vi "OpenG Reverse 2D Array Template.vi"() -> ()   [LabVIEW 2012]
panel:
  in  "by rows or columns (rows)":enum16{"rows", "columns"}(ring)
  in  "Array":dbl[][](array[numeric]) format="%.2f"
  out "Reversed Array":dbl[][](array[numeric]) format="%.2f"
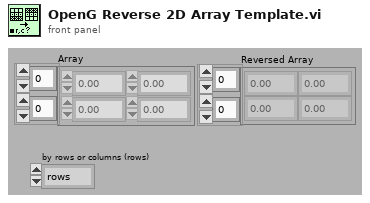
[diagram p1: front panel]
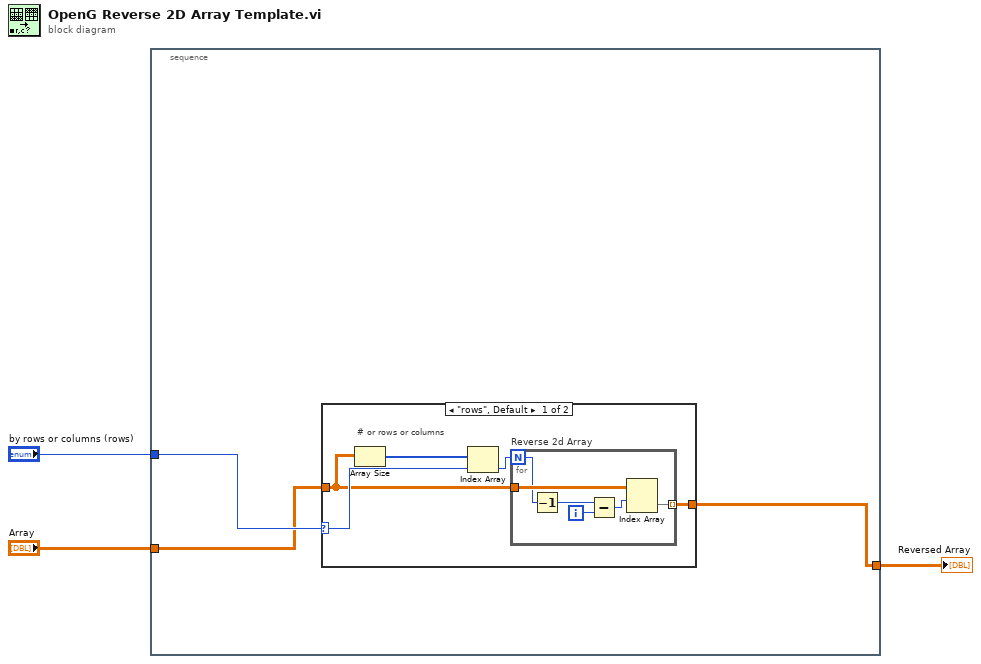
[diagram p0: block diagram]
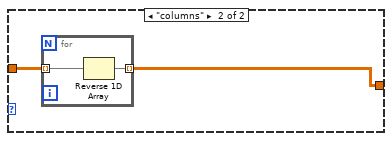
[diagram p2: hidden frame]
diagram:
  n1 = stacked-sequence {
    tunnel: "Array" -> [w5]
    tunnel: "by rows or columns (rows)" -> [w6]
    tunnel: [w4] -> w1
    frame #0 {
      n2 = case shown="\"rows\", Default" w6 {
        selector: w6 -> [w9 _]
        tunnel: w5 -> [w8 w19]
        tunnel: [w7 w18] -> w4
        frame "rows", Default {
          # "# or rows or columns"
          n3 = Array Size(array=w8) -> (size(s)=w11:i32[])
          n4 = Index Array(array=w11, index=w9) -> (element=w10:i32)
          n5 = for "Reverse 2d Array" {
            N: w10 -> [w16]
            tunnel: w8 -> [w17]
            tunnel: [w12] -> w7 mode=indexing
            i -> [w14]
            n6 = Decrement(x=w16) -> (x-1=w15:i32)
            n7 = Subtract(x=w15, y=w14) -> (x-y=w13:i32)
            n8 = Index Array(array=w17, index (row)=w13) -> (element=w12:dbl[])  [unwired: 1 in]
          }
        }
        frame "columns" {
          n9 = for {
            tunnel: w19 -> [w21] mode=indexing
            tunnel: [w20] -> w18 mode=indexing
            n10 = Reverse 1D Array(array=w21) -> (reversed array=w20:dbl[])
          }
        }
      }
    }
  }
  "Reversed Array" <- w1
